vi "flattenPressureToXML.vi"   [LabVIEW 2012, in "UnitsAndXML.lvlib"]
doc: "Generates an XML string for <B>pressure</B> in the unit specified in <B>pressureUnitInXML</B>. Connect <B>pressure</B> and <B>pressureAgain</B> to the same source. The VI uses <B>pressureAgain</B> to obtain the data name."
uses:
  <userlib>/Common/UnitsAndXML/UnitsAndXML.lvlib
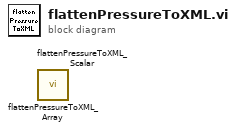
[diagram p0: block diagram]
diagram:
  n1 = call <userlib>:"flattenPressureToXML_Array.vi"() -> ()  [unwired: 10 in, 2 out]
  n2 = call <userlib>:"flattenPressureToXML_Scalar.vi"() -> ()  [unwired: 10 in, 2 out]
